vi "Steps_to_Add.vi"(11 "Cluster":T1) -> (2 "logical AND":bool, 3 "output cluster":T1={"Current Position"=[-1, -1, 0], "Steps Increment"=[-1, -1, 0], "Steps to Add "=[-1, -1, 0], "Final Position"=[-1, -1, 0]})   [LabVIEW 2018]
uses:
  Steps.ctl
  <vilib>/Analysis/2dsp.llb/Real FFT.vi
  <vilib>/Analysis/NI_AALPro.lvlib
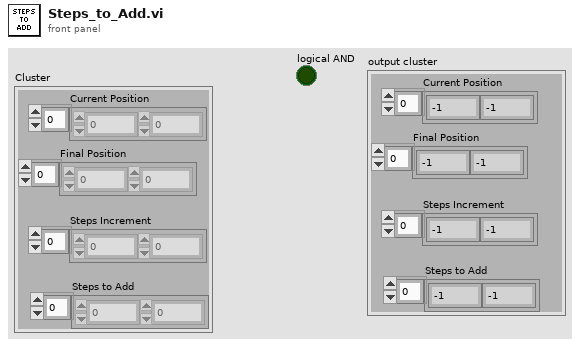
[diagram p1: front panel]
types:
  T1 = typedef "Steps.ctl" = cluster{"Current Position":i32[], "Steps Increment":i32[], "Steps to Add ":i32[], "Final Position":i32[]}
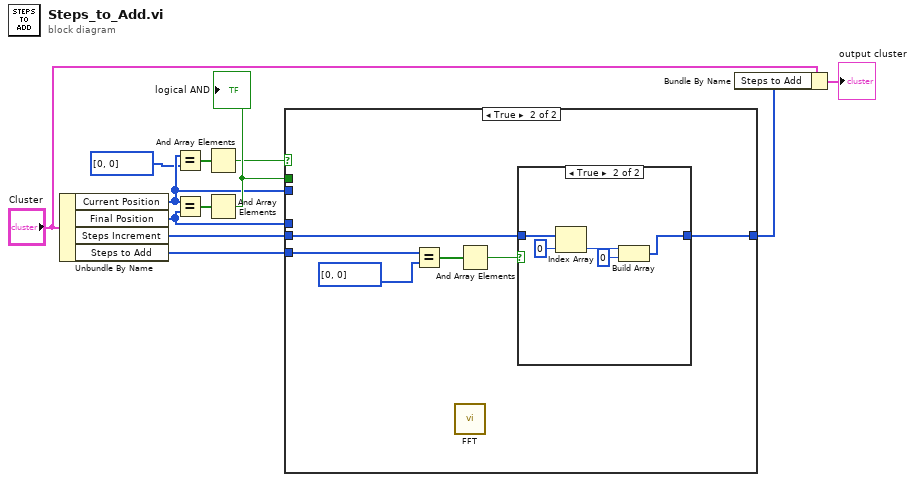
[diagram p0: block diagram]
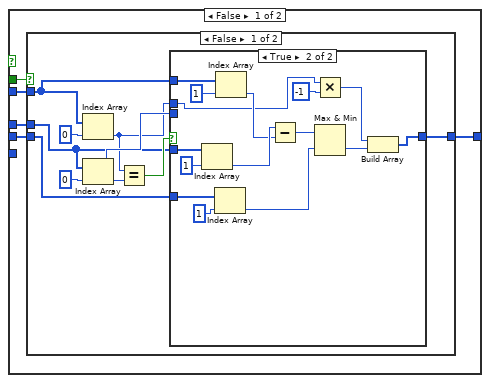
[diagram p2: hidden frame]
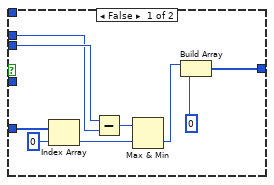
[diagram p3: hidden frame]
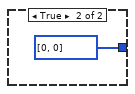
[diagram p4: hidden frame]
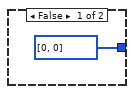
[diagram p5: hidden frame]
diagram:
  n1 = Unbundle By Name("Cluster") -> ("Current Position"=w4:i32[], "Final Position"=w9:i32[], "Steps Increment"=w10:i32[], "Steps to Add"=w1:i32[])
  n2 = Equal?(x=w4, y=i32[] [0, 0]) -> (x = y?=w5:bool[])
  n3 = Equal?(x=w4, y=w9) -> (x = y?=w12:bool[])
  n4 = And Array Elements(Boolean array=w5) -> (logical AND=w2:bool)
  n5 = And Array Elements(Boolean array=w12) -> (logical AND=w11:bool)
  "logical AND" <- w11
  n6 = case shown="True" w2 {
    tunnel: w11 -> [w13 _]
    tunnel: w10 -> [w16 w53]
    tunnel: w9 -> [w17 _]
    tunnel: [w14 w52] -> w8
    tunnel: w4 -> [w15 _]
    tunnel: w1 -> [_ w55]
    frame False {
      n7 = case shown="False" w13 {
        tunnel: w17 -> [w19 _]
        tunnel: w16 -> [w23 _]
        tunnel: w15 -> [w18 _]
        tunnel: [w20 i32[] [0, 0]] -> w14
        frame False {
          n8 = Index Array(array=w18, index=0) -> (element=w21:i32)
          n9 = Index Array(array=w19, index=0) -> (element=w22:i32)
          n10 = Equal?(x=w21, y=w22) -> (x = y?=w24:bool)
          n11 = case shown="True" w24 {
            tunnel: w23 -> [w34 w45]
            tunnel: w22 -> [w31 _]
            tunnel: w21 -> [w30 w39]
            tunnel: [w28 w43] -> w20
            tunnel: w19 -> [_ w50]
            tunnel: w18 -> [_ w42]
            frame False {
              n12 = Index Array(array=w34, index=0) -> (element=w32:i32)
              n13 = Subtract(x=w31, y=w30) -> (x-y=w33:i32)
              n14 = Max & Min(x=w33, y=w32) -> (min(x,y)=w29:i32)  [unwired: 1 out]
              n15 = Build Array(w29, 0 ("element")) -> (w28:i32[])
            }
            frame True {
              n16 = Index Array(array=w50, index=1) -> (element=w48:i32)
              n17 = Index Array(array=w45, index=1) -> (element=w44:i32)
              n18 = Index Array(array=w42, index=1) -> (element=w40:i32)
              n19 = Subtract(x=w48, y=w40) -> (x-y=w47:i32)
              n20 = Multiply(x=w39, y=-1) -> (x*y=w36:i32)
              n21 = Max & Min(x=w47, y=w44) -> (min(x,y)=w37:i32)  [unwired: 1 out]
              n22 = Build Array(w36, w37) -> (w43:i32[])
            }
          }
        }
        frame True {
        }
      }
    }
    frame True {
      n23 = Equal?(x=w55, y=i32[] [0, 0]) -> (x = y?=w57:bool[])
      n24 = call-poly <vilib>:"FFT.vi"() -> ()  [unwired: 10 in, 2 out]
      n25 = And Array Elements(Boolean array=w57) -> (logical AND=w54:bool)
      n26 = case shown="True" w54 {
        tunnel: [i32[] [0, 0] ("Steps Increment") w59] -> w52
        tunnel: w53 -> [_ w63]
        frame False {
        }
        frame True {
          n27 = Index Array(array=w63, index=0) -> (element=w61:i32)
          n28 = Build Array(w61, 0 ("element")) -> (w59:i32[])
        }
      }
    }
  }
  n29 = Bundle By Name(cluster="Cluster", "Steps to Add"=w8) -> (→"output cluster":T1)
